vi "car_Timer_main.vi"(7 "Command (Check Timer)":T1=enum."Check Timer", 8 "error in (no error)":errorcluster, 10 "Pause":bool, 11 "Target Time (s)":dbl) -> (0 "error out":errorcluster, 3 "Elapsed":bool)   [LabVIEW 2009]
doc: "This VI is the main VI for the Timer module. This VI runs a Timer that compares the time from when the Timer was started to the Target Time in seconds.\n\nThis Timer can be paused. When the Timer is paused an offset is calculated and stored in memory."
uses:
  car_Timer_Command_enum.ctl
panel:
  # "Inputs"
  # "Outputs"
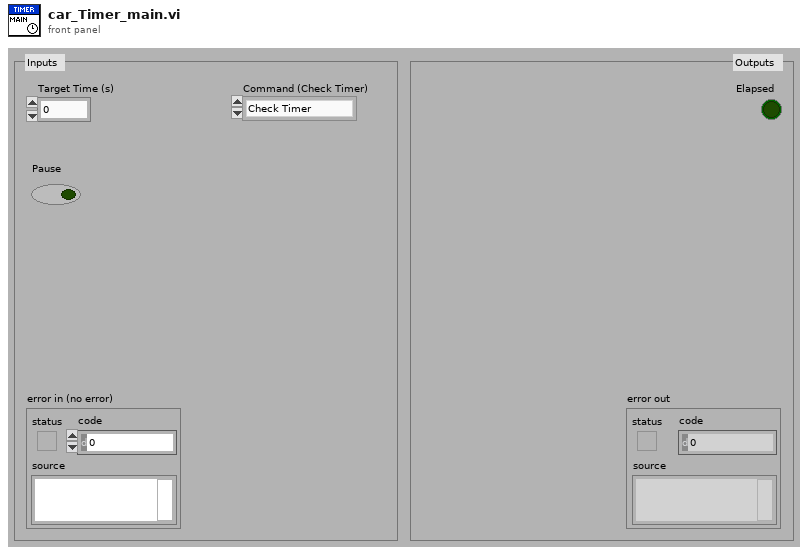
[diagram p1: front panel]
types:
  T1 = typedef "car_Timer_Command_enum.ctl" = enum16{"Start Timer", "Check Timer"}
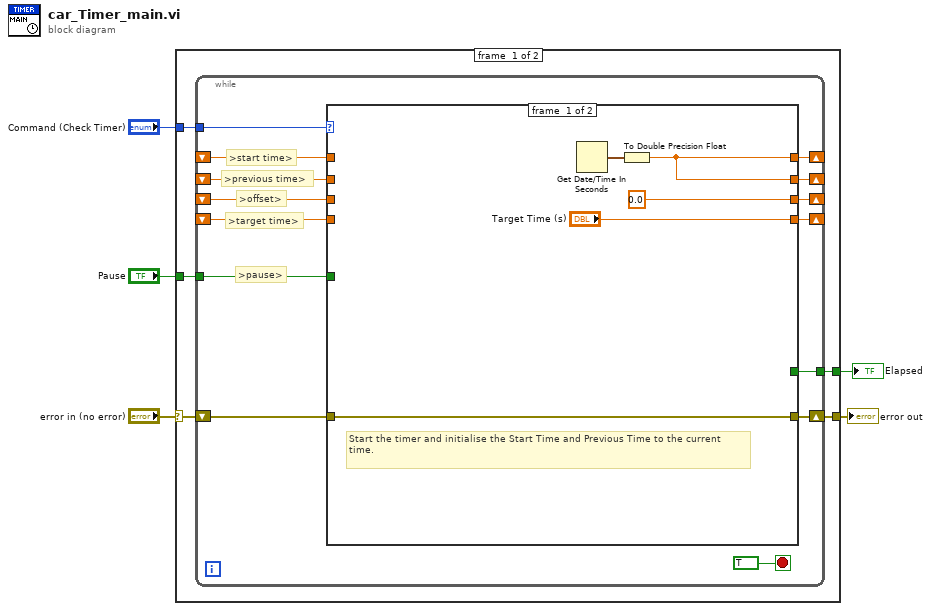
[diagram p0: block diagram]
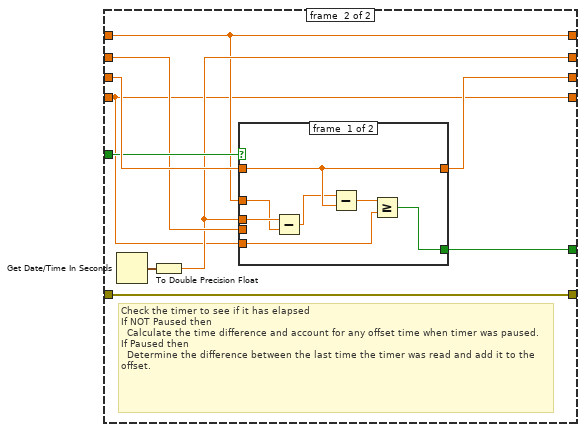
[diagram p2: hidden frame]
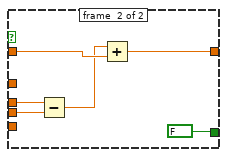
[diagram p3: hidden frame]
diagram:
  n1 = case shown="No Error" "error in (no error)" {
    selector: "error in (no error)" -> [w10 w53]
    tunnel: [w9 w53] -> w4
    tunnel: "Command (Check Timer)" -> [w8 _]
    tunnel: "Pause" -> [w7 _]
    tunnel: [w6 _] -> w1
    frame #0 {
      n2 = while {
        shift-right: [w23] -> w9
        shift-left: w10 -> [w24]
        tunnel: w8 -> [w22]
        tunnel: w7 -> [w21]
        shift-right: [w19] -> _
        shift-left: _ -> [w20]
        shift-right: [w17] -> _
        shift-left: _ -> [w18]
        tunnel: [w15] -> w6
        shift-right: [w14] -> _
        shift-left: _ -> [w13]
        shift-right: [w11] -> _
        shift-left: _ -> [w12]
        stop <- TRUE stop-if-true
        # ">previous time>"
        # ">pause>"
        # ">target time>"
        # ">offset>"
        # ">start time>"
        n3 = case shown="\"Start Timer\"" w22 {
          tunnel: w24 -> [w29 w39]
          tunnel: [w29 w39] -> w23
          tunnel: w21 -> [_ w37]
          tunnel: w20 -> [_ w31]
          tunnel: [w26 w31] -> w19
          tunnel: w18 -> [_ w38]
          tunnel: [0.0 w34] -> w17
          tunnel: [_ w36] -> w15
          tunnel: [w26 w32] -> w14
          tunnel: w13 -> [_ w33]
          tunnel: w12 -> [_ w30]
          tunnel: ["Target Time (s)" w30] -> w11
          frame #0 {
            # "Start the timer and initialise the Start Time and Previous Time to the current time."
            n4 = Get Date/Time In Seconds() -> (seconds since 1Jan1904=w28:timestamp)
            n5 = To Double Precision Float(number=w28) -> (double precision float=w26:dbl)
          }
          frame #1 {
            # "Check the timer to see if it has elapsed\nIf NOT Paused then \n  Calculate the time difference and account for any offset time when timer was paused.\nIf Paused then\n  Determine the difference between the last time the timer was read and add it to the offset."
            n6 = Get Date/Time In Seconds() -> (seconds since 1Jan1904=w35:timestamp)
            n7 = To Double Precision Float(number=w35) -> (double precision float=w32:dbl)
            n8 = case shown="False" w37 {
              tunnel: w38 -> [w44 w50]
              tunnel: [w45 FALSE] -> w36
              tunnel: [w44 w51] -> w34
              tunnel: w30 -> [w46 _]
              tunnel: w33 -> [_ w49]
              tunnel: w32 -> [w43 w48]
              tunnel: w31 -> [w42 _]
              frame #0 {
                n9 = Subtract(x=w43, y=w42) -> (x-y=w41:dbl)
                n10 = Subtract(x=w41, y=w44) -> (x-y=w40:dbl)
                n11 = Greater Or Equal?(x=w40, y=w46) -> (x >= y?=w45:bool)
              }
              frame #1 {
                n12 = Subtract(x=w48, y=w49) -> (x-y=w47:dbl)
                n13 = Add(x=w47, y=w50) -> (x+y=w51:dbl)
              }
            }
          }
        }
      }
    }
    frame #1 {
    }
  }
  "error out" <- w4
  "Elapsed" <- w1
